vi "SR1.ProcCases.vi"(0 "i ref in":refnum<vi>, 1 "selector":string, 2 "Data":T1, 3 "call cluster":T2={"Object"="", "Selector"="", "CallType"=enum."synchronous", "Async Object"="", "Async Selector"="", "Data Descriptor"="", "Data"=[], "Error #"=0, "Expire"=0}, 5 "error in (no error)":errorcluster) -> (14 "i ref out":refnum<vi>, 17 "answer cluster":T2={"Object"="", "Selector"="", "CallType"=enum."synchronous", "Async Object"="", "Async Selector"="", "Data Descriptor"="", "Data"=[], "Error #"=0, "Expire"=0}, 19 "error out":errorcluster)   [LabVIEW 2014, in "SR1.lvlib"]
doc: "This method is called by a process from within the default case in the event loop. The methods of a class that are linked to events will be called from THIS method. Add your code here."
uses:
  SR1.lvlib
  CS_Core/CSSystem/CoreDefs/CoreDefs.call_type.ctl
  CS_Core/BaseProcess/BaseProcess.descriptor string definition.ctl
  CS_Core/CSSystem/CoreDefs/CoreDefs.rawDataType.ctl
  CS_Core/CSSystem/CoreLib/CoreLib.string 2 byte array.vi
  CS_Core/CSSystem/CoreLib/CoreLib.double 2 byte array.vi
  CS_Core/CSSystem/CoreLib/CoreLib.byte array 2 double.vi
  CS_Core/CSSystem/CoreLib/CoreLib.int 2 byte array.vi
  CS_Core/CSSystem/CoreLib/CoreLib.byte array 2 int.vi
  CS_Core/CSSystem/CoreLib/CoreLib.lvlib
  CS_Core/BaseProcess/BaseProcess.lvlib
  CS_Core/CSApplicationBaseClasses/DeviceBase/DeviceBase.lvlib
  CS_Core/CSApplicationBaseClasses/NABase/NABase.lvlib
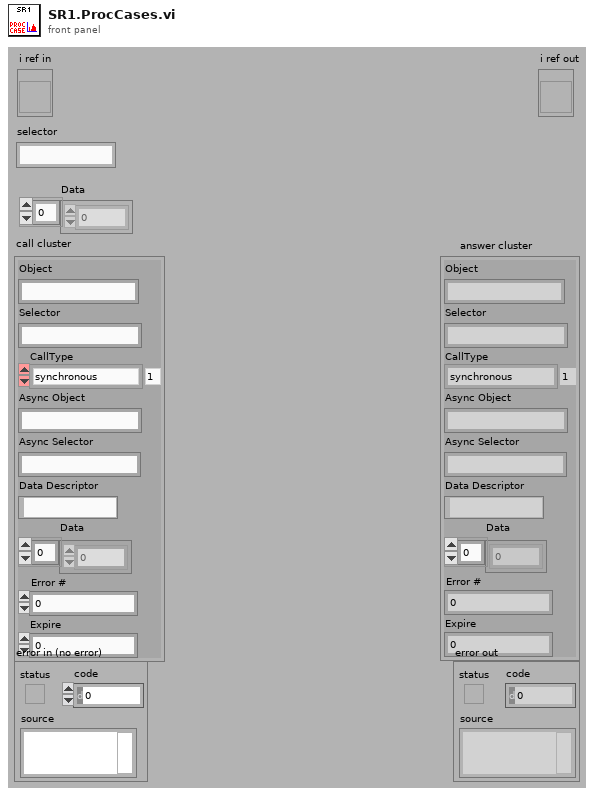
[diagram p1: front panel]
types:
  T1 = typedef "CoreDefs.rawDataType.ctl" = i8[]
  T2 = typedef "CoreDefs.call_type.ctl" = cluster{"Object":string, "Selector":string, "CallType":enum16{"simple", "synchronous", "asynchronous"}, "Async Object":string, "Async Selector":string, "Data Descriptor":T3, "Data":T1, "Error #":i32, "Expire":u32}
  T3 = typedef "BaseProcess.lvlib/BaseProcess.descriptor string definition.ctl" = string
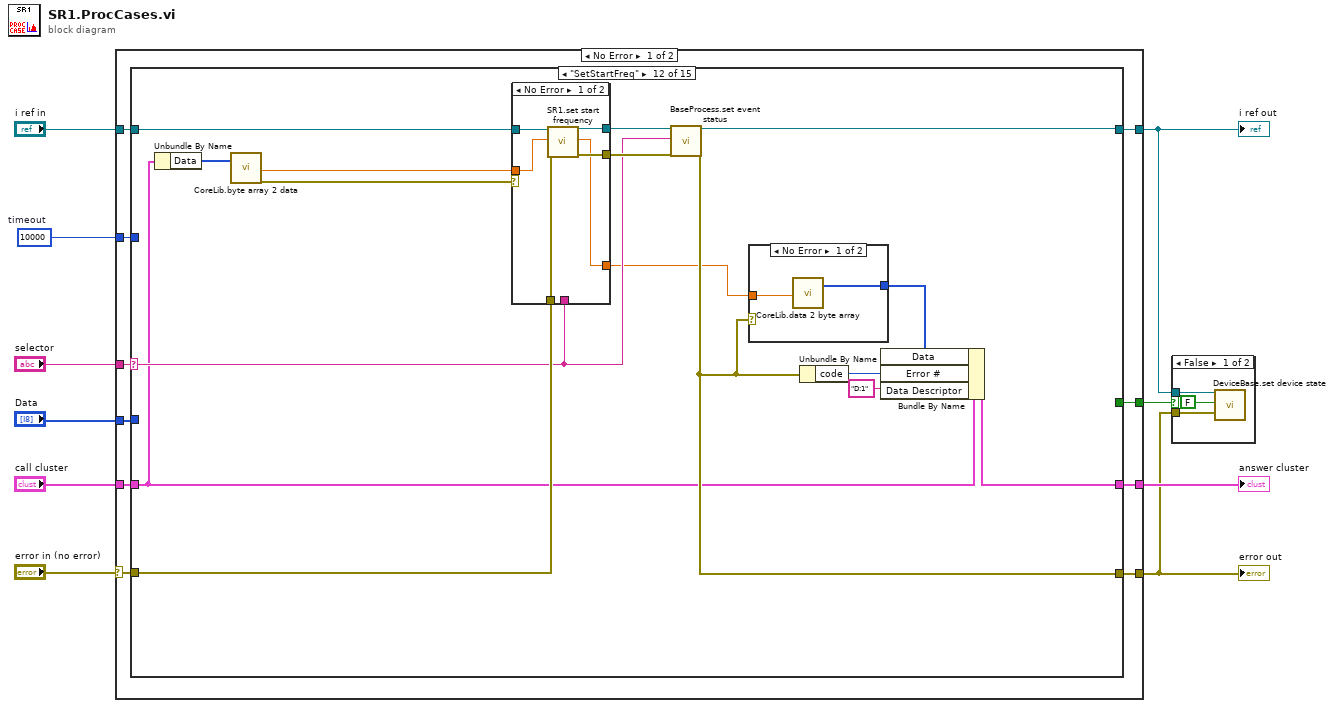
[diagram p0: block diagram]
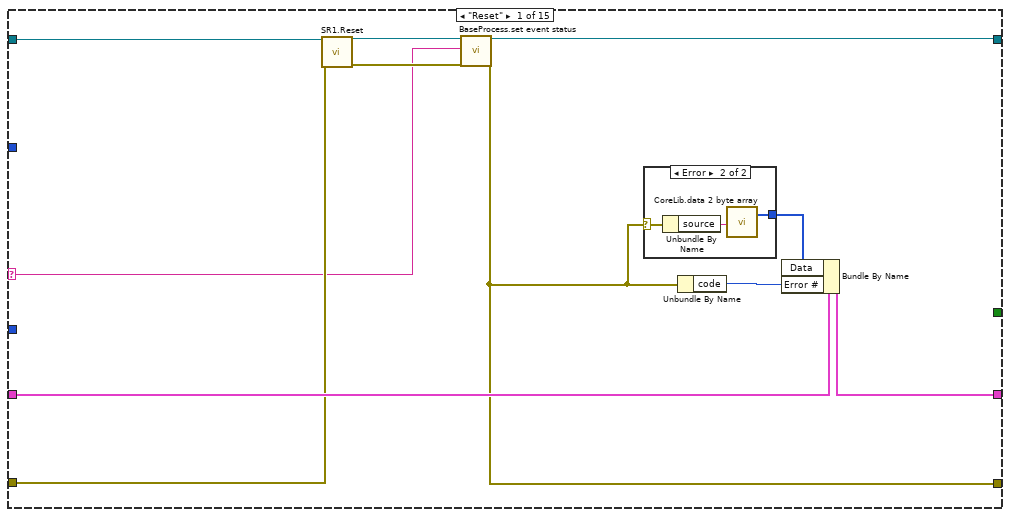
[diagram p2: hidden frame]
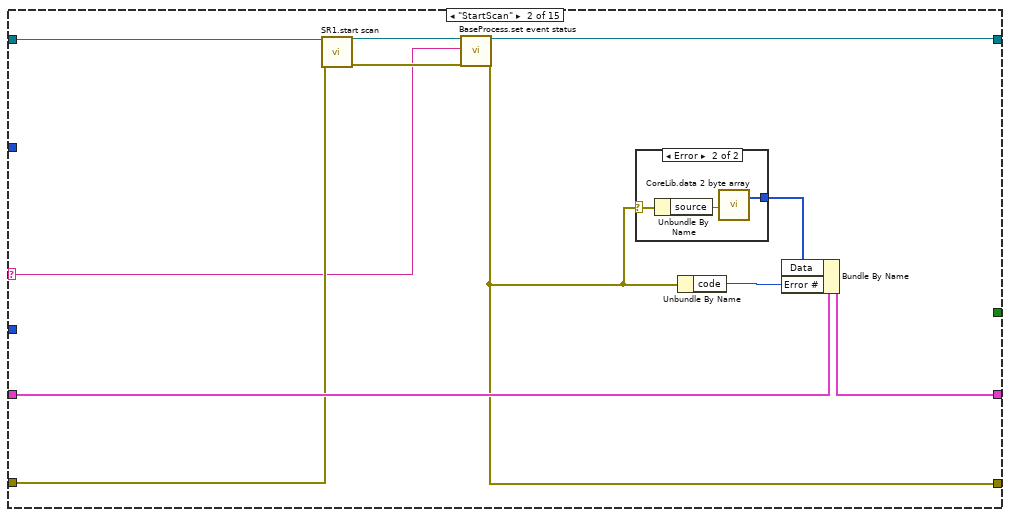
[diagram p4: hidden frame]
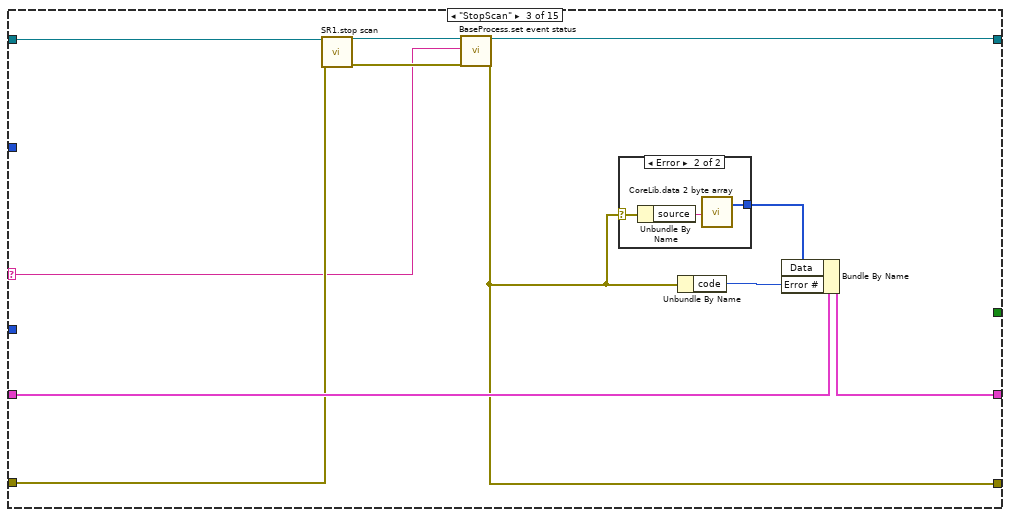
[diagram p6: hidden frame]
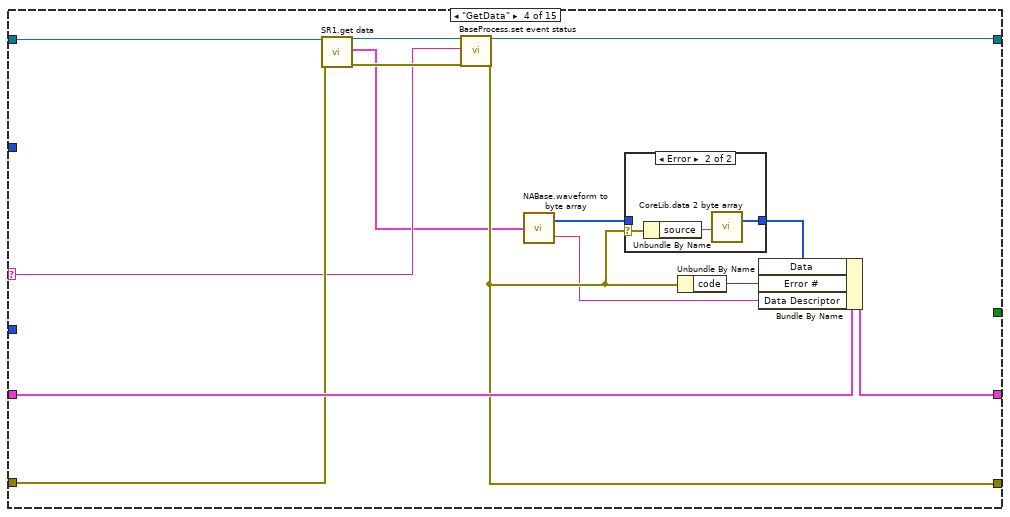
[diagram p8: hidden frame]
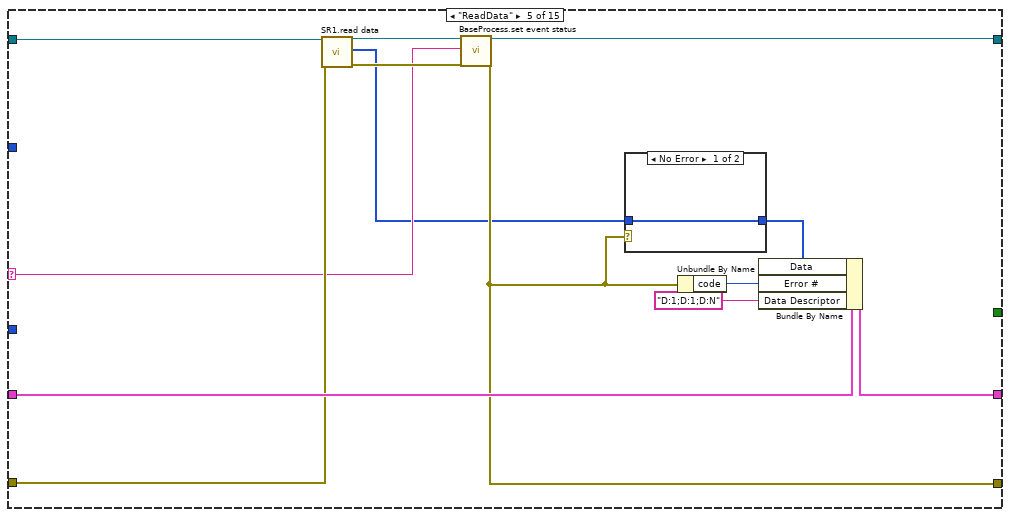
[diagram p10: hidden frame]
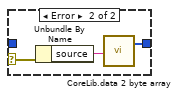
[diagram p11: hidden frame]
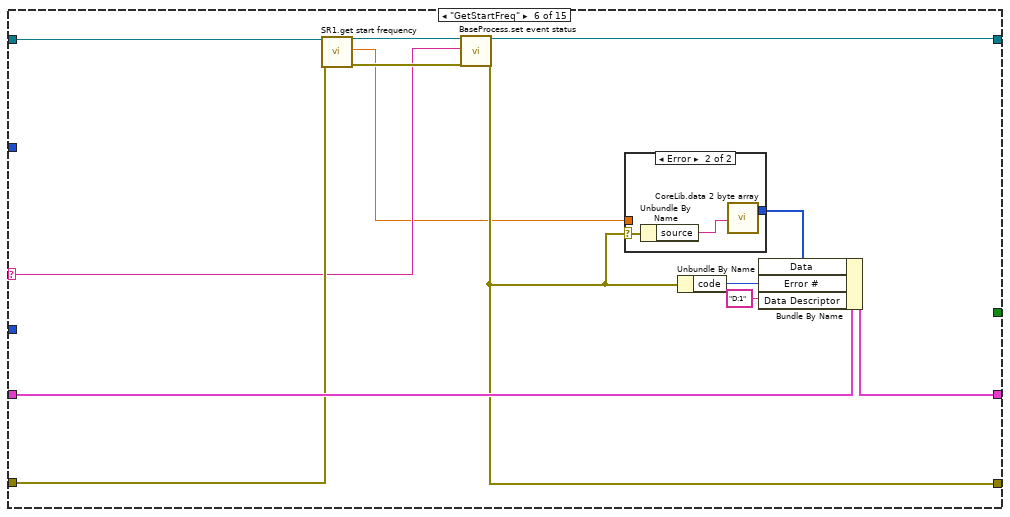
[diagram p12: hidden frame]
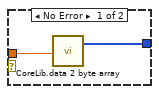
[diagram p13: hidden frame]
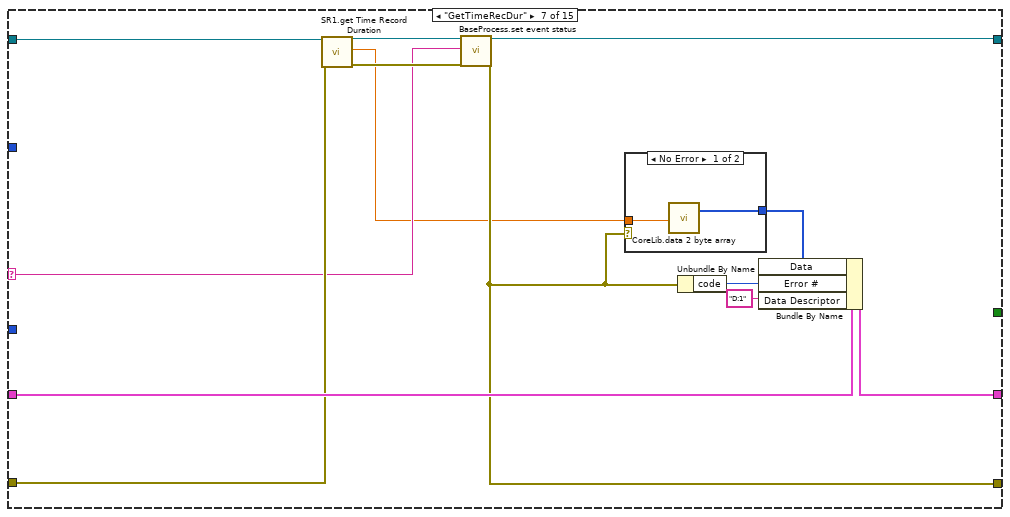
[diagram p14: hidden frame]
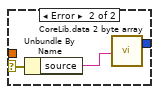
[diagram p15: hidden frame]
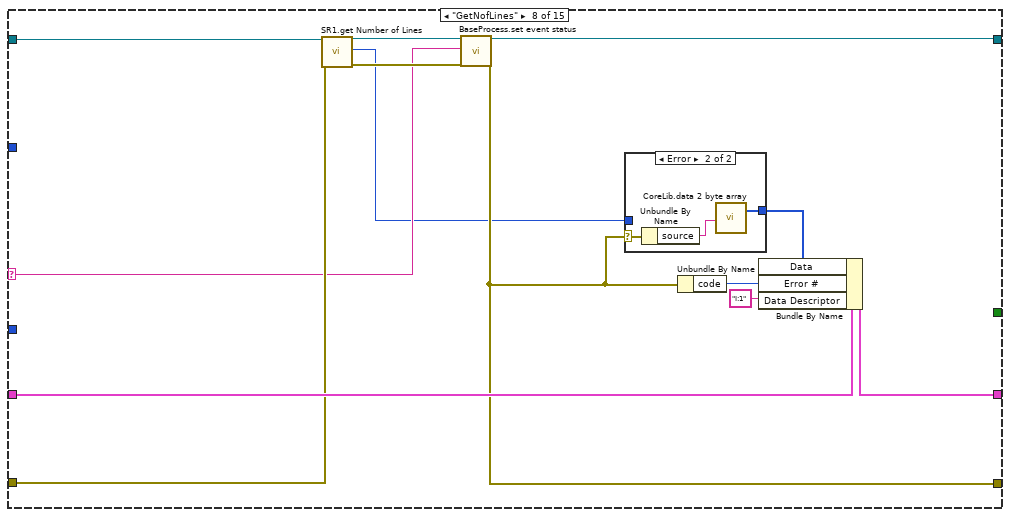
[diagram p16: hidden frame]
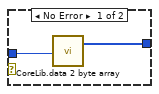
[diagram p17: hidden frame]
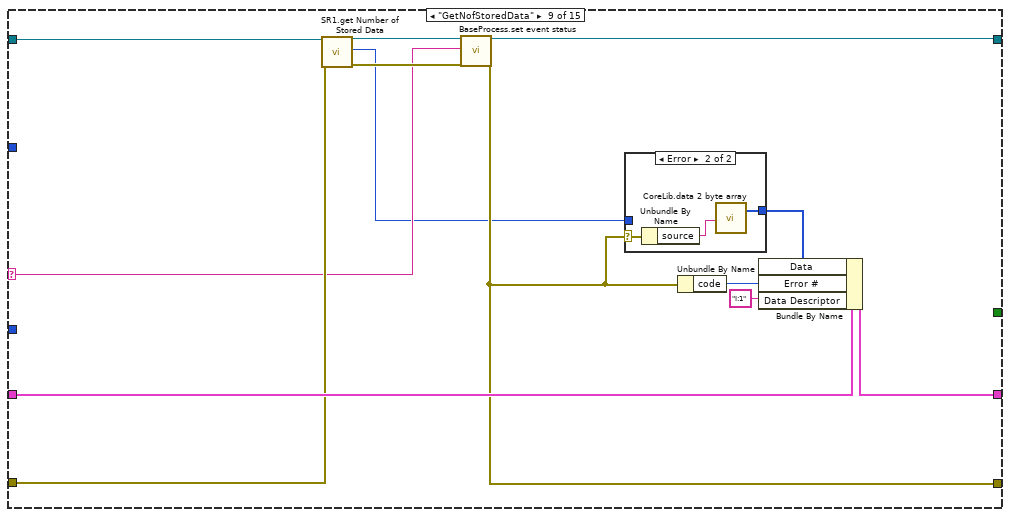
[diagram p18: hidden frame]
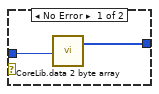
[diagram p19: hidden frame]
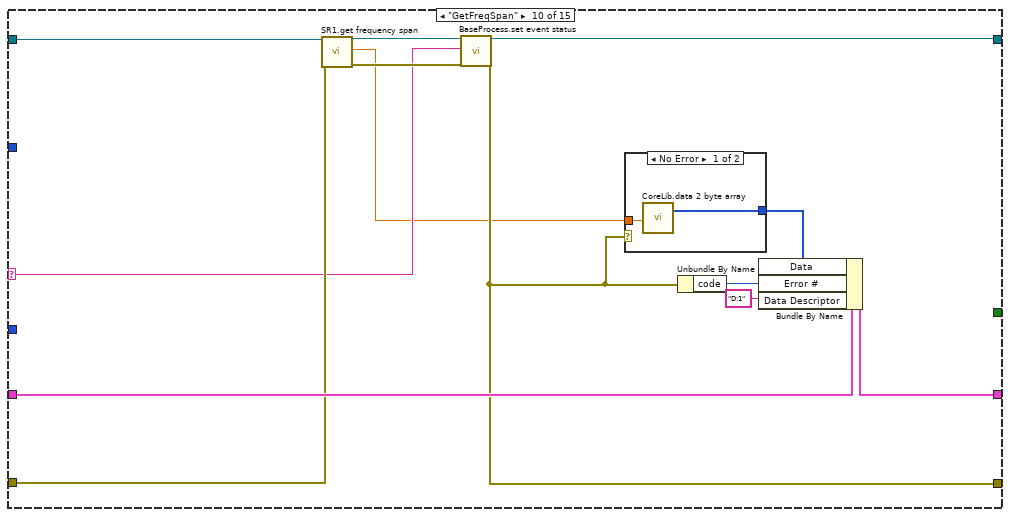
[diagram p20: hidden frame]
diagram:
  w5 = 10000  # timeout
  n1 = case shown="No Error" "error in (no error)" {
    selector: "error in (no error)" -> [w11 w306]
    tunnel: "selector" -> [w20 _]
    tunnel: [w19 w307] -> w9
    tunnel: "Data" -> [w18 _]
    tunnel: "call cluster" -> [w17 w307]
    tunnel: "i ref in" -> [w16 w308]
    tunnel: w5 -> [w15 _]
    tunnel: [w14 w306] -> w4
    tunnel: [w13 w308] -> w3
    tunnel: [w12 _] -> w2
    frame No Error {
      n2 = case shown="\"SetStartFreq\"" w20 {
        selector: w20 -> [w21 w37 w51 w66 w83 w100 w118 w136 w154 w172 w191 w208 w241 w274 w298]
        tunnel: w18 -> [_ _ _ _ _ _ _ _ _ _ _ _ _ _ w299]
        tunnel: w16 -> [w27 w42 w56 w72 w89 w106 w124 w142 w160 w178 w196 w214 w247 w279 w305]
        tunnel: [w24 w39 w53 w69 w86 w103 w121 w139 w157 w175 w193 w211 w244 w276 w304] -> w13
        tunnel: w17 -> [w31 w45 w59 w76 w93 w110 w128 w146 w164 w182 w190 w207 w240 w273 w300]
        tunnel: [w30 w44 w58 w75 w92 w109 w127 w145 w163 w181 w198 w217 w250 w281 w301] -> w19
        tunnel: w11 -> [w26 w41 w55 w71 w88 w105 w123 w141 w159 w177 w195 w213 w246 w278 w303]
        tunnel: [w22 w36 w50 w67 w84 w101 w119 w137 w155 w173 w189 w209 w242 w268 w302] -> w14
        tunnel: w15 -> [_ _ _ _ _ _ _ _ _ _ _ _ w237 _ _]
        tunnel: [_ _ _ _ _ _ _ _ _ _ _ _ _ _ TRUE] -> w12
        frame "Reset" {
          n3 = call "SR1.Reset.vi"("i ref in"=w27, "error in (no error)"=w26) -> ("i ref out"=w25:refnum<vi>, "error out"=w23:errorcluster)  [unwired: 16 in]
          n4 = call "BaseProcess.set event status.vi"("i ref in"=w25, "EventStatus"=w21, "error in (no error)"=w23) -> ("i ref out"=w24:refnum<vi>, "error out"=w22:errorcluster)  [unwired: 14 in, 1 out]
          n5 = case shown="Error" w22 {
            selector: w22 -> [_ w34]
            tunnel: [_ w32] -> w28
            frame No Error {
            }
            frame Error {
              n6 = Unbundle By Name(w34) -> ("source"=w33:string)
              n7 = call-poly "CoreLib.data 2 byte array.vi"("string"=w33) -> ("byteArray out"=w32:T1)  [unwired: 18 in]
            }
          }
          n8 = Unbundle By Name(w22) -> ("code"=w29:i32)
          n9 = Bundle By Name(cluster=w31, "Data"=w28, "Error #"=w29) -> (w30:T2)
        }
        frame "StartScan" {
          n10 = call "SR1.start scan.vi"("i ref in"=w42, "error in (no error)"=w41) -> ("i ref out"=w40:refnum<vi>, "error out"=w38:errorcluster)  [unwired: 16 in]
          n11 = call "BaseProcess.set event status.vi"("i ref in"=w40, "EventStatus"=w37, "error in (no error)"=w38) -> ("i ref out"=w39:refnum<vi>, "error out"=w36:errorcluster)  [unwired: 14 in, 1 out]
          n12 = case shown="Error" w36 {
            selector: w36 -> [_ w48]
            tunnel: [_ w46] -> w35
            frame No Error {
            }
            frame Error {
              n13 = Unbundle By Name(w48) -> ("source"=w47:string)
              n14 = call-poly "CoreLib.data 2 byte array.vi"("string"=w47) -> ("byteArray out"=w46:T1)  [unwired: 18 in]
            }
          }
          n15 = Unbundle By Name(w36) -> ("code"=w43:i32)
          n16 = Bundle By Name(cluster=w45, "Data"=w35, "Error #"=w43) -> (w44:T2)
        }
        frame "StopScan" {
          n17 = call "SR1.stop scan.vi"("i ref in"=w56, "error in (no error)"=w55) -> ("i ref out"=w54:refnum<vi>, "error out"=w52:errorcluster)  [unwired: 16 in]
          n18 = call "BaseProcess.set event status.vi"("i ref in"=w54, "EventStatus"=w51, "error in (no error)"=w52) -> ("i ref out"=w53:refnum<vi>, "error out"=w50:errorcluster)  [unwired: 14 in, 1 out]
          n19 = case shown="Error" w50 {
            selector: w50 -> [_ w62]
            tunnel: [_ w60] -> w49
            frame No Error {
            }
            frame Error {
              n20 = Unbundle By Name(w62) -> ("source"=w61:string)
              n21 = call-poly "CoreLib.data 2 byte array.vi"("string"=w61) -> ("byteArray out"=w60:T1)  [unwired: 18 in]
            }
          }
          n22 = Unbundle By Name(w50) -> ("code"=w57:i32)
          n23 = Bundle By Name(cluster=w59, "Data"=w49, "Error #"=w57) -> (w58:T2)
        }
        frame "GetData" {
          n24 = call "SR1.get data.vi"("i ref in"=w72, "error in (no error)"=w71) -> ("i ref out"=w70:refnum<vi>, "Output Waveform"=w65:cluster{dbl, dbl, dbl[]}, "error out"=w68:errorcluster)  [unwired: 15 in]
          n25 = call "BaseProcess.set event status.vi"("i ref in"=w70, "EventStatus"=w66, "error in (no error)"=w68) -> ("i ref out"=w69:refnum<vi>, "error out"=w67:errorcluster)  [unwired: 14 in, 1 out]
          n26 = call "NABase.waveform to byte array.vi"("Waveform"=w65) -> ("byteArray out"=w64:T1, "dataDescriptor"=w63:string)
          n27 = case shown="Error" w67 {
            selector: w67 -> [_ w80]
            tunnel: [w77 w79] -> w73
            tunnel: w64 -> [w77 _]
            frame No Error {
            }
            frame Error {
              n28 = Unbundle By Name(w80) -> ("source"=w78:string)
              n29 = call-poly "CoreLib.data 2 byte array.vi"("string"=w78) -> ("byteArray out"=w79:T1)  [unwired: 18 in]
            }
          }
          n30 = Unbundle By Name(w67) -> ("code"=w74:i32)
          n31 = Bundle By Name(cluster=w76, "Data"=w73, "Error #"=w74, "Data Descriptor"=w63) -> (w75:T2)
        }
        frame "ReadData" {
          n32 = call "SR1.read data.vi"("i ref in"=w89, "error in (no error)"=w88) -> ("i ref out"=w87:refnum<vi>, "Output Waveform"=w82:T1, "error out"=w85:errorcluster)  [unwired: 15 in]
          n33 = call "BaseProcess.set event status.vi"("i ref in"=w87, "EventStatus"=w83, "error in (no error)"=w85) -> ("i ref out"=w86:refnum<vi>, "error out"=w84:errorcluster)  [unwired: 14 in, 1 out]
          n34 = case shown="No Error" w84 {
            selector: w84 -> [_ w97]
            tunnel: [w94 w96] -> w90
            tunnel: w82 -> [w94 _]
            frame No Error {
            }
            frame Error {
              n35 = Unbundle By Name(w97) -> ("source"=w95:string)
              n36 = call-poly "CoreLib.data 2 byte array.vi"("string"=w95) -> ("byteArray out"=w96:T1)  [unwired: 18 in]
            }
          }
          n37 = Unbundle By Name(w84) -> ("code"=w91:i32)
          n38 = Bundle By Name(cluster=w93, "Data"=w90, "Error #"=w91, "Data Descriptor"="D:1;D:1;D:N") -> (w92:T2)
        }
        frame "GetStartFreq" {
          n39 = call "SR1.get start frequency.vi"("i ref in"=w106, "error in (no error)"=w105) -> ("i ref out"=w104:refnum<vi>, "Start Frequency"=w99:dbl, "error out"=w102:errorcluster)  [unwired: 15 in]
          n40 = call "BaseProcess.set event status.vi"("i ref in"=w104, "EventStatus"=w100, "error in (no error)"=w102) -> ("i ref out"=w103:refnum<vi>, "error out"=w101:errorcluster)  [unwired: 14 in, 1 out]
          n41 = case shown="Error" w101 {
            selector: w101 -> [_ w115]
            tunnel: [w111 w113] -> w107
            tunnel: w99 -> [w112 _]
            frame No Error {
              n42 = call-poly "CoreLib.data 2 byte array.vi"("f64"=w112) -> ("byteArray out"=w111:T1)  [unwired: 18 in]
            }
            frame Error {
              n43 = Unbundle By Name(w115) -> ("source"=w114:string)
              n44 = call-poly "CoreLib.data 2 byte array.vi"("string"=w114) -> ("byteArray out"=w113:T1)  [unwired: 18 in]
            }
          }
          n45 = Unbundle By Name(w101) -> ("code"=w108:i32)
          n46 = Bundle By Name(cluster=w110, "Data"=w107, "Error #"=w108, "Data Descriptor"="D:1") -> (w109:T2)
        }
        frame "GetTimeRecDur" {
          n47 = call "SR1.get Time Record Duration.vi"("i ref in"=w124, "error in (no error)"=w123) -> ("i ref out"=w122:refnum<vi>, "TimeRecordDuration[s]"=w117:dbl, "error out"=w120:errorcluster)  [unwired: 15 in]
          n48 = call "BaseProcess.set event status.vi"("i ref in"=w122, "EventStatus"=w118, "error in (no error)"=w120) -> ("i ref out"=w121:refnum<vi>, "error out"=w119:errorcluster)  [unwired: 14 in, 1 out]
          n49 = case shown="No Error" w119 {
            selector: w119 -> [_ w133]
            tunnel: [w129 w131] -> w125
            tunnel: w117 -> [w130 _]
            frame No Error {
              n50 = call-poly "CoreLib.data 2 byte array.vi"("f64"=w130) -> ("byteArray out"=w129:T1)  [unwired: 18 in]
            }
            frame Error {
              n51 = Unbundle By Name(w133) -> ("source"=w132:string)
              n52 = call-poly "CoreLib.data 2 byte array.vi"("string"=w132) -> ("byteArray out"=w131:T1)  [unwired: 18 in]
            }
          }
          n53 = Unbundle By Name(w119) -> ("code"=w126:i32)
          n54 = Bundle By Name(cluster=w128, "Data"=w125, "Error #"=w126, "Data Descriptor"="D:1") -> (w127:T2)
        }
        frame "GetNofLines" {
          n55 = call "SR1.get Number of Lines.vi"("i ref in"=w142, "error in (no error)"=w141) -> ("i ref out"=w140:refnum<vi>, "NofLines"=w135:i32, "error out"=w138:errorcluster)  [unwired: 15 in]
          n56 = call "BaseProcess.set event status.vi"("i ref in"=w140, "EventStatus"=w136, "error in (no error)"=w138) -> ("i ref out"=w139:refnum<vi>, "error out"=w137:errorcluster)  [unwired: 14 in, 1 out]
          n57 = case shown="Error" w137 {
            selector: w137 -> [_ w151]
            tunnel: [w147 w150] -> w143
            tunnel: w135 -> [w148 _]
            frame No Error {
              n58 = call-poly "CoreLib.data 2 byte array.vi"("i32"=w148) -> ("byteArray out"=w147:T1)  [unwired: 18 in]
            }
            frame Error {
              n59 = Unbundle By Name(w151) -> ("source"=w149:string)
              n60 = call-poly "CoreLib.data 2 byte array.vi"("string"=w149) -> ("byteArray out"=w150:T1)  [unwired: 18 in]
            }
          }
          n61 = Unbundle By Name(w137) -> ("code"=w144:i32)
          n62 = Bundle By Name(cluster=w146, "Data"=w143, "Error #"=w144, "Data Descriptor"="I:1") -> (w145:T2)
        }
        frame "GetNofStoredData" {
          n63 = call "SR1.get Number of Stored Data.vi"("i ref in"=w160, "error in (no error)"=w159) -> ("i ref out"=w158:refnum<vi>, "NofStoredData"=w153:i32, "error out"=w156:errorcluster)  [unwired: 15 in]
          n64 = call "BaseProcess.set event status.vi"("i ref in"=w158, "EventStatus"=w154, "error in (no error)"=w156) -> ("i ref out"=w157:refnum<vi>, "error out"=w155:errorcluster)  [unwired: 14 in, 1 out]
          n65 = case shown="Error" w155 {
            selector: w155 -> [_ w169]
            tunnel: [w165 w168] -> w161
            tunnel: w153 -> [w166 _]
            frame No Error {
              n66 = call-poly "CoreLib.data 2 byte array.vi"("i32"=w166) -> ("byteArray out"=w165:T1)  [unwired: 18 in]
            }
            frame Error {
              n67 = Unbundle By Name(w169) -> ("source"=w167:string)
              n68 = call-poly "CoreLib.data 2 byte array.vi"("string"=w167) -> ("byteArray out"=w168:T1)  [unwired: 18 in]
            }
          }
          n69 = Unbundle By Name(w155) -> ("code"=w162:i32)
          n70 = Bundle By Name(cluster=w164, "Data"=w161, "Error #"=w162, "Data Descriptor"="I:1") -> (w163:T2)
        }
        frame "GetFreqSpan" {
          n71 = call "SR1.get frequency span.vi"("i ref in"=w178, "error in (no error)"=w177) -> ("i ref out"=w176:refnum<vi>, "FreqSpan [Hz]"=w171:dbl, "error out"=w174:errorcluster)  [unwired: 15 in]
          n72 = call "BaseProcess.set event status.vi"("i ref in"=w176, "EventStatus"=w172, "error in (no error)"=w174) -> ("i ref out"=w175:refnum<vi>, "error out"=w173:errorcluster)  [unwired: 14 in, 1 out]
          n73 = case shown="No Error" w173 {
            selector: w173 -> [_ w187]
            tunnel: [w183 w186] -> w179
            tunnel: w171 -> [w184 _]
            frame No Error {
              n74 = call-poly "CoreLib.data 2 byte array.vi"("f64"=w184) -> ("byteArray out"=w183:T1)  [unwired: 18 in]
            }
            frame Error {
              n75 = Unbundle By Name(w187) -> ("source"=w185:string)
              n76 = call-poly "CoreLib.data 2 byte array.vi"("string"=w185) -> ("byteArray out"=w186:T1)  [unwired: 18 in]
            }
          }
          n77 = Unbundle By Name(w173) -> ("code"=w180:i32)
          n78 = Bundle By Name(cluster=w182, "Data"=w179, "Error #"=w180, "Data Descriptor"="D:1") -> (w181:T2)
        }
        frame "Init" {
          n79 = call "SR1.init.vi"("i ref in"=w196, "error in (no error)"=w195) -> ("i ref out"=w194:refnum<vi>, "error out"=w192:errorcluster)  [unwired: 16 in]
          n80 = call "BaseProcess.set event status.vi"("i ref in"=w194, "EventStatus"=w191, "error in (no error)"=w192) -> ("i ref out"=w193:refnum<vi>, "error out"=w189:errorcluster)  [unwired: 14 in, 1 out]
          n81 = case shown="Error" w189 {
            selector: w189 -> [_ w201]
            tunnel: [_ w199] -> w188
            frame No Error {
            }
            frame Error {
              n82 = Unbundle By Name(w201) -> ("source"=w200:string)
              n83 = call-poly "CoreLib.data 2 byte array.vi"("string"=w200) -> ("byteArray out"=w199:T1)  [unwired: 18 in]
            }
          }
          n84 = Unbundle By Name(w189) -> ("code"=w197:i32)
          n85 = Bundle By Name(cluster=w190, "Data"=w188, "Error #"=w197) -> (w198:T2)
        }
        frame "SetStartFreq" {
          n86 = Unbundle By Name(w207) -> ("Data"=w206:T1)
          n87 = call-poly "CoreLib.byte array 2 data.vi"("byteArray"=w206) -> ("d64"=w204:dbl, "error out"=w203:errorcluster)  [unwired: 16 in, 1 out]
          n88 = case shown="No Error" w203 {
            tunnel: w214 -> [w223 w225]
            tunnel: w213 -> [w222 w227]
            tunnel: [w221 w225] -> w212
            tunnel: [w220 w228] -> w210
            tunnel: w208 -> [_ w226]
            tunnel: w204 -> [w219 _]
            tunnel: [w218 0.0 ("act bin width")] -> w205
            frame No Error {
              n89 = call "SR1.set start frequency.vi"("i ref in"=w223, "Start Frequency"=w219, "error in (no error)"=w222) -> ("i ref out"=w221:refnum<vi>, "Start Frequency"=w218:dbl, "error out"=w220:errorcluster)  [unwired: 14 in]
            }
            frame Error {
              n90 = call "CoreLib.set data type mismatch.vi"("error in (no error)"=w227, "error source"=w226) -> ("error out"=w228:errorcluster)  [unwired: 17 in]
            }
          }
          n91 = call "BaseProcess.set event status.vi"("i ref in"=w212, "EventStatus"=w208, "error in (no error)"=w210) -> ("i ref out"=w211:refnum<vi>, "error out"=w209:errorcluster)  [unwired: 14 in, 1 out]
          n92 = case shown="No Error" w209 {
            selector: w209 -> [_ w233]
            tunnel: [w229 w232] -> w215
            tunnel: w205 -> [w230 _]
            frame No Error {
              n93 = call-poly "CoreLib.data 2 byte array.vi"("f64"=w230) -> ("byteArray out"=w229:T1)  [unwired: 18 in]
            }
            frame Error {
              n94 = Unbundle By Name(w233) -> ("source"=w231:string)
              n95 = call-poly "CoreLib.data 2 byte array.vi"("string"=w231) -> ("byteArray out"=w232:T1)  [unwired: 18 in]
            }
          }
          n96 = Unbundle By Name(w209) -> ("code"=w216:i32)
          n97 = Bundle By Name(cluster=w207, "Data"=w215, "Error #"=w216, "Data Descriptor"="D:1") -> (w217:T2)
        }
        frame "SetNofLines" {
          n98 = Unbundle By Name(w240) -> ("Data"=w239:T1)
          n99 = call-poly "CoreLib.byte array 2 data.vi"("byteArray"=w239) -> ("i32"=w236:i32, "error out"=w235:errorcluster)  [unwired: 16 in, 1 out]
          n100 = case shown="No Error" w235 {
            tunnel: w247 -> [w255 w257]
            tunnel: w246 -> [w254 w259]
            tunnel: [w253 w257] -> w245
            tunnel: [w252 w260] -> w243
            tunnel: w241 -> [_ w258]
            tunnel: w236 -> [w251 _]
            tunnel: [w251 0 ("act bin width")] -> w238
            tunnel: w237 -> [_ _]
            frame No Error {
              n101 = call "SR1.set Number of Lines.vi"("i ref in"=w255, "NofLines"=w251, "error in (no error)"=w254) -> ("i ref out"=w253:refnum<vi>, "error out"=w252:errorcluster)  [unwired: 15 in]
            }
            frame Error {
              n102 = call "CoreLib.set data type mismatch.vi"("error in (no error)"=w259, "error source"=w258) -> ("error out"=w260:errorcluster)  [unwired: 17 in]
            }
          }
          n103 = call "BaseProcess.set event status.vi"("i ref in"=w245, "EventStatus"=w241, "error in (no error)"=w243) -> ("i ref out"=w244:refnum<vi>, "error out"=w242:errorcluster)  [unwired: 14 in, 1 out]
          n104 = case shown="No Error" w242 {
            selector: w242 -> [_ w265]
            tunnel: [w261 w264] -> w248
            tunnel: w238 -> [w262 _]
            frame No Error {
              n105 = call-poly "CoreLib.data 2 byte array.vi"("i32"=w262) -> ("byteArray out"=w261:T1)  [unwired: 18 in]
            }
            frame Error {
              n106 = Unbundle By Name(w265) -> ("source"=w263:string)
              n107 = call-poly "CoreLib.data 2 byte array.vi"("string"=w263) -> ("byteArray out"=w264:T1)  [unwired: 18 in]
            }
          }
          n108 = Unbundle By Name(w242) -> ("code"=w249:i32)
          n109 = Bundle By Name(cluster=w240, "Data"=w248, "Error #"=w249, "Data Descriptor"="I:1") -> (w250:T2)
        }
        frame "SetFreqSpan" {
          n110 = Unbundle By Name(w273) -> ("Data"=w272:T1)
          n111 = call-poly "CoreLib.byte array 2 data.vi"("byteArray"=w272) -> ("d64"=w271:dbl, "error out"=w270:errorcluster)  [unwired: 16 in, 1 out]
          n112 = case shown="No Error" w270 {
            tunnel: w279 -> [w292 w293]
            tunnel: w278 -> [w291 w295]
            tunnel: [w290 w293] -> w277
            tunnel: [w289 w296] -> w275
            tunnel: w274 -> [_ w294]
            tunnel: w271 -> [w288 _]
            tunnel: [w287 _] -> w266
            frame No Error {
              n113 = call "SR1.set frequency span.vi"("i ref in"=w292, "FreqSpan [Hz]"=w288, "error in (no error)"=w291) -> ("i ref out"=w290:refnum<vi>, "FreqSpan [Hz]"=w287:dbl, "error out"=w289:errorcluster)  [unwired: 14 in]
            }
            frame Error {
              n114 = call "CoreLib.set data type mismatch.vi"("error in (no error)"=w295, "error source"=w294) -> ("error out"=w296:errorcluster)  [unwired: 17 in]
            }
          }
          n115 = call "BaseProcess.set event status.vi"("i ref in"=w277, "EventStatus"=w274, "error in (no error)"=w275) -> ("i ref out"=w276:refnum<vi>, "error out"=w268:errorcluster)  [unwired: 14 in, 1 out]
          n116 = case shown="No Error" w268 {
            selector: w268 -> [_ w286]
            tunnel: [w283 w284] -> w269
            tunnel: w266 -> [w282 _]
            frame No Error {
              n117 = call-poly "CoreLib.data 2 byte array.vi"("f64"=w282) -> ("byteArray out"=w283:T1)  [unwired: 18 in]
            }
            frame Error {
              n118 = Unbundle By Name(w286) -> ("source"=w285:string)
              n119 = call-poly "CoreLib.data 2 byte array.vi"("string"=w285) -> ("byteArray out"=w284:T1)  [unwired: 18 in]
            }
          }
          n120 = Unbundle By Name(w268) -> ("code"=w280:i32)
          n121 = Bundle By Name(cluster=w273, "Data"=w269, "Error #"=w280, "Data Descriptor"=T3 "D:1") -> (w281:T2)
        }
        frame Default {
          n122 = call "NABase.ProcCases.vi"("i ref in"=w305, "selector"=w298, "Data"=w299, "call cluster"=w300, "error in (no error)"=w303) -> ("i ref out"=w304:refnum<vi>, "answer cluster"=w301:T2, "error out"=w302:errorcluster)  [unwired: 12 in]
        }
      }
    }
    frame Error {
    }
  }
  "answer cluster" <- w9
  "i ref out" <- w3
  "error out" <- w4
  n123 = case shown="False" w2 {
    tunnel: w4 -> [w311 _]
    tunnel: w3 -> [w310 _]
    frame False {
      n124 = call "DeviceBase.set device state.vi"("i ref in"=w310, "implicit"=FALSE, "device error"=w311) -> ()  [unwired: 14 in, 3 out]
    }
    frame True {
    }
  }
